vi "半加器电路实验.vi"() -> ()   [LabVIEW 2018]
panel:
  in  "结束":bool
  out "进位C":bool
  out "和数S":bool
  in  "加数B":bool
  in  "被加数A":bool
  # "74HC00：与非门"
  # "74HC04：非门"
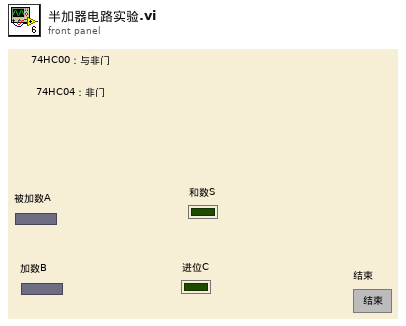
[diagram p1: front panel]
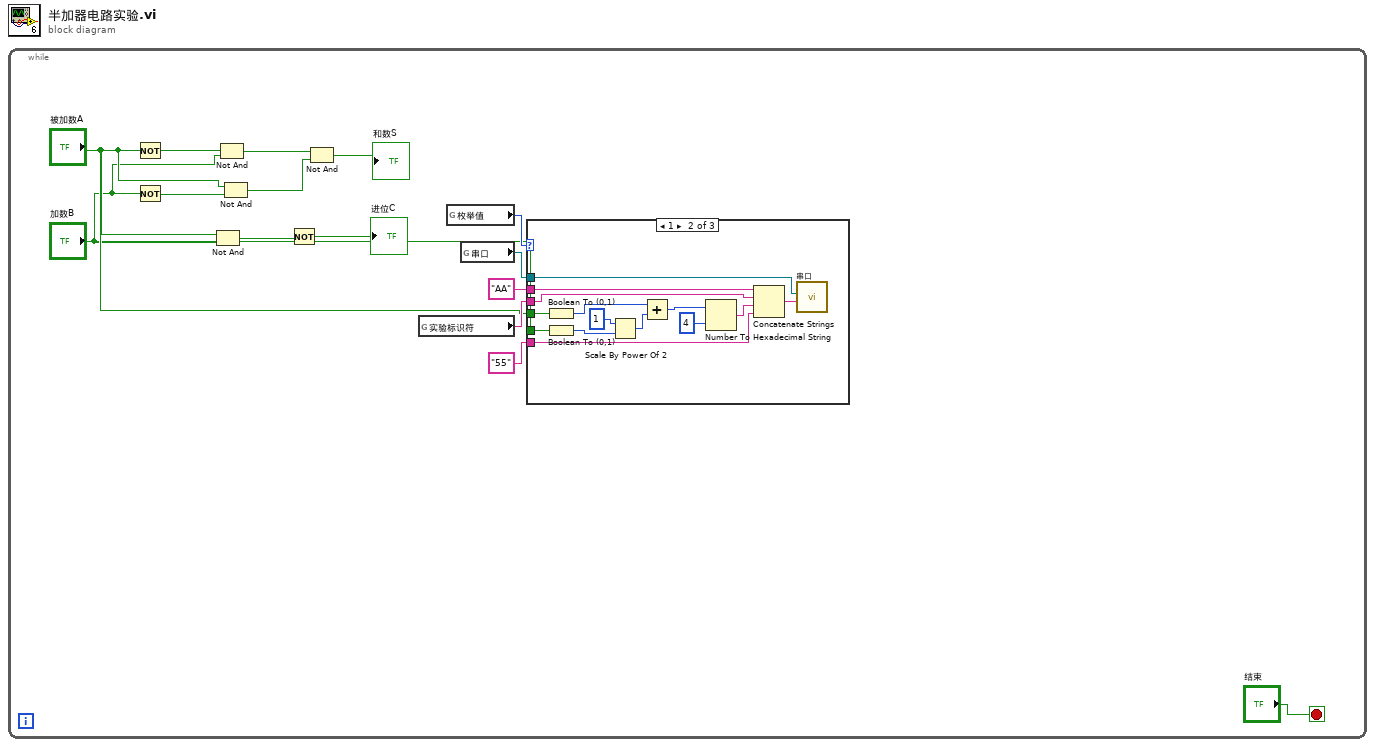
[diagram p0: block diagram]
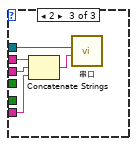
[diagram p3: hidden frame]
diagram:
  n1 = while {
    stop <- "结束" stop-if-true
    n2 = Not(x="被加数A") -> (.not. x?=w15:bool)
    n3 = Not(x="加数B") -> (.not. x?=w14:bool)
    n4 = Not And(1:"加数B", 2:"被加数A") -> (0:w9:bool)
    n5 = Not And(1:"加数B", 2:w15) -> (0:w13:bool)
    n6 = Not And(1:w14, 2:"被加数A") -> (0:w12:bool)
    n7 = Not(x=w9) -> (.not. x?=→"进位C":bool)
    n8 = Not And(1:w12, 2:w13) -> (0:→"和数S":bool)
    n9 = global read "全局变量.vi" "实验标识符"() -> (w5:string)
    n10 = global read "全局变量.vi" "枚举值"() -> (w7:i8)
    n11 = global read "全局变量.vi" "串口"() -> (w6:refnum<visa-resource-name>)
    n12 = case shown="1" w7 {
      tunnel: "加数B" -> [_ w24 _]
      tunnel: "被加数A" -> [_ w23 _]
      tunnel: w6 -> [_ w22 w32]
      tunnel: w5 -> [_ w21 w33]
      tunnel: "55" -> [_ w20 w30]
      tunnel: "AA" -> [_ w19 w31]
      frame 0, Default {
      }
      frame 1 {
        n13 = Boolean To (0,1)(Boolean=w23) -> (0, 1=w28:i16)
        n14 = Boolean To (0,1)(Boolean=w24) -> (0, 1=w26:i16)
        n15 = Scale By Power Of 2(n=1, x=w26) -> (x*2^n=w27:i16)
        n16 = Add(x=w28, y=w27) -> (x+y=w18:i16)
        n17 = Number To Hexadecimal String(1:4, 2:w18) -> (0:w16:string)
        n18 = Concatenate Strings(w19, w21, w16, w20) -> (w29:string)
        n19 = call "串口.vi"("字符串"=w29, "VISA resource name"=w22) -> ()  [unwired: 10 in]
      }
      frame 2 {
        n20 = Concatenate Strings(w31, w33, w30) -> (w34:string)
        n21 = call "串口.vi"("字符串"=w34, "VISA resource name"=w32) -> ()  [unwired: 10 in]
      }
    }
  }
